vi "Insert_FileName_In_Error.vi"(3 "error in":errorcluster, 4 "Path":path) -> (5 "error out":errorcluster)   [LabVIEW 2018]
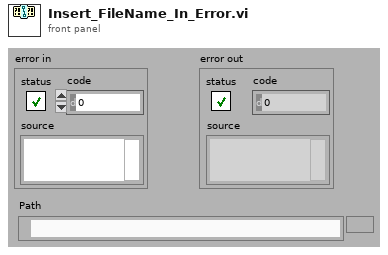
[diagram p1: front panel]
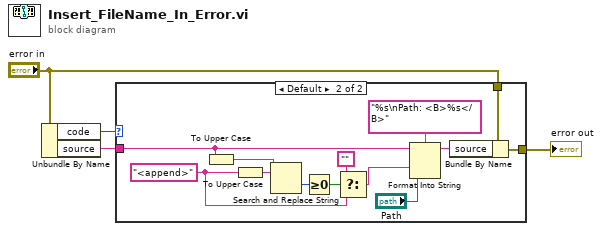
[diagram p0: block diagram]
diagram:
  n1 = Unbundle By Name("error in") -> ("code"=w1:i32, "source"=w4:string)
  n2 = case shown="Default" w1 {
    tunnel: w4 -> [_ w18]
    tunnel: "error in" -> [w5 w17]
    tunnel: [w5 w16] -> w2
    frame 0 {
    }
    frame Default {
      w9 = "<append>" ("search string")
      n3 = To Upper Case(1:w18) -> (0:w6:string)
      n4 = To Upper Case(1:w9) -> (0:w7:string)
      n5 = Search and Replace String(input string=w6, search string=w7) -> (offset past replacement=w11:i32)  [unwired: 6 in, 3 out]
      n6 = Greater Or Equal To 0?(x=w11) -> (x >= 0?=w12:bool)
      n7 = Select(t="", s=w12, f=w9) -> (s? t:f=w8:string)
      n8 = Format Into String(format string="%s\nPath: <B>%s</B>", initial string=w18, w8, "Path") -> (resulting string=w13:string)  [unwired: 1 in, 1 out]
      n9 = Bundle By Name(cluster=w17, "source"=w13) -> (w16:errorcluster)
    }
  }
  "error out" <- w2
